vi "CheckCarPos.vi"(8 "Car Position":u8, 9 "Current Step":i8) -> (3 "Position Ok?":bool)   [LabVIEW 2019]
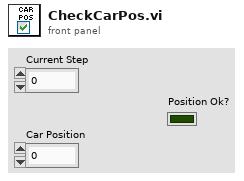
[diagram p1: front panel]
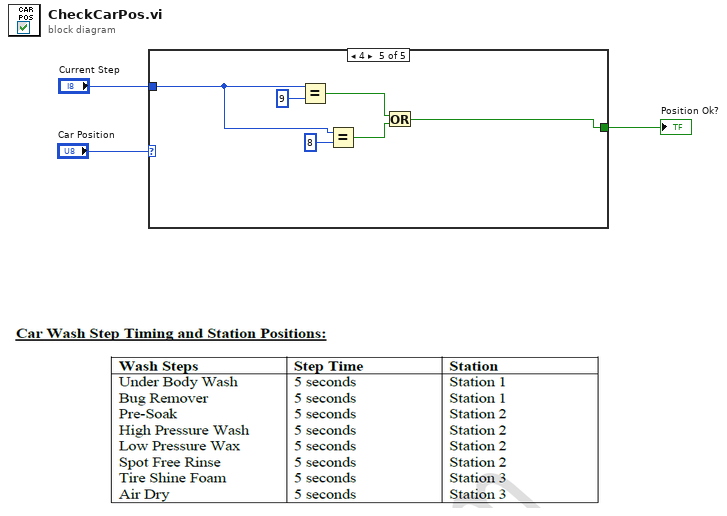
[diagram p0: block diagram]
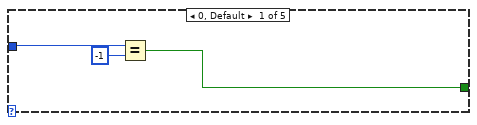
[diagram p2: hidden frame]
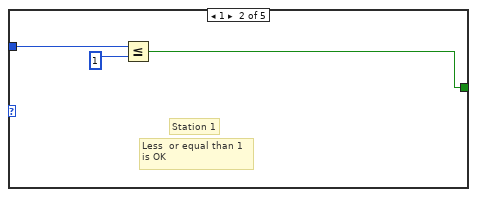
[diagram p3: hidden frame]
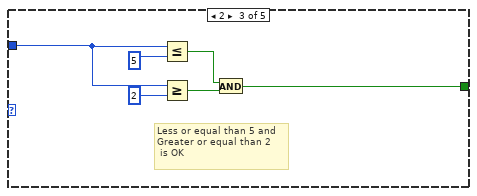
[diagram p4: hidden frame]
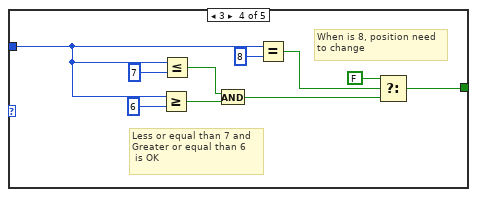
[diagram p5: hidden frame]
diagram:
  n1 = case shown="4" "Car Position" {
    tunnel: "Current Step" -> [w5 w8 w12 w17 w29]
    tunnel: [w6 w7 w10 w19 w26] -> w1
    frame 0, Default {
      n2 = Equal?(x=w5, y=i8 -1) -> (x = y?=w6:bool)
    }
    frame 1 {
      # "Less  or equal than 1 \nis OK"
      # "Station 1"
      n3 = Less Or Equal?(x=w8, y=u8 1) -> (x <= y?=w7:bool)
    }
    frame 2 {
      # "Less or equal than 5 and \nGreater or equal than 2\n is OK"
      n4 = Less Or Equal?(x=w12, y=u8 5) -> (x <= y?=w13:bool)
      n5 = Greater Or Equal?(x=w12, y=u8 2) -> (x >= y?=w14:bool)
      n6 = And(x=w13, y=w14) -> (x .and. y?=w10:bool)
    }
    frame 3 {
      # "When is 8, position need\nto change"
      # "Less or equal than 7 and \nGreater or equal than 6\n is OK"
      n7 = Greater Or Equal?(x=w17, y=u8 6) -> (x >= y?=w24:bool)
      n8 = Less Or Equal?(x=w17, y=u8 7) -> (x <= y?=w22:bool)
      n9 = And(x=w22, y=w24) -> (x .and. y?=w18:bool)
      n10 = Equal?(x=w17, y=i8 8) -> (x = y?=w20:bool)
      n11 = Select(t=FALSE, s=w20, f=w18) -> (s? t:f=w19:bool)
    }
    frame 4 {
      n12 = Equal?(x=w29, y=i8 9) -> (x = y?=w27:bool)
      n13 = Equal?(x=w29, y=i8 8) -> (x = y?=w28:bool)
      n14 = Or(x=w27, y=w28) -> (x .or. y?=w26:bool)
    }
  }
  "Position Ok?" <- w1
